vi "Stop Cooking.vi"(8 "error in (no error)":errorcluster, 11 "Cooker Actor in":refnum<class "Cooker Actor.lvclass">) -> (0 "error out":errorcluster, 3 "Cooker Actor out":refnum<class "Cooker Actor.lvclass">)   [LabVIEW 2021, in "Cooker Actor.lvlib" / "Cooker Actor.lvclass"]
uses:
  Cooker Actor.lvclass
  Oven Actor/Oven Actor Messages/Stop Heat Msg/Stop Heat Msg.lvclass
  <vilib>/ActorFramework/Actor/Actor.lvclass
  Cooker Actor Messages/Update Cooker Duration Msg/Update Cooker Duration Msg.lvclass
  Kitchen Actor Messages/Dye Whole Recipe Table Msg/Dye Whole Recipe Table Msg.lvclass
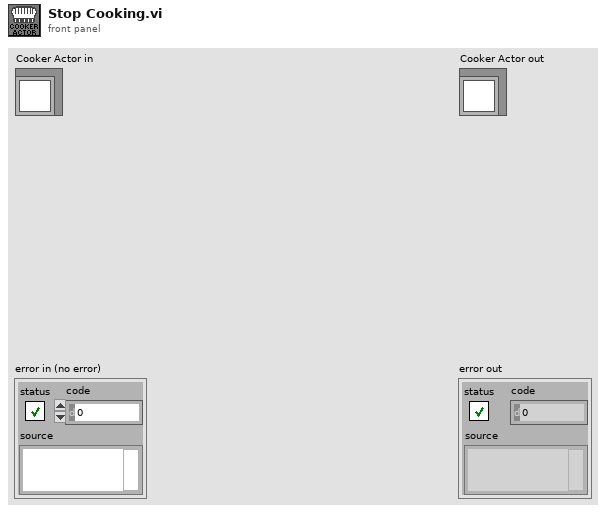
[diagram p1: front panel]
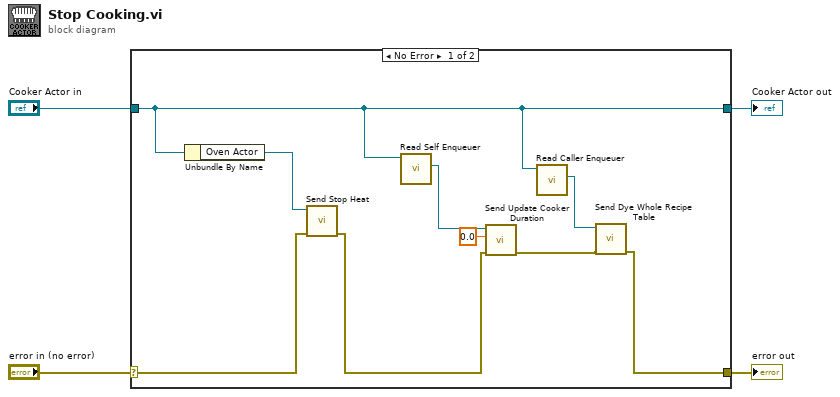
[diagram p0: block diagram]
diagram:
  n1 = case shown="No Error" "error in (no error)" {
    selector: "error in (no error)" -> [w12 w15]
    tunnel: [w5 w15] -> w3
    tunnel: [w8 w14] -> w1
    tunnel: "Cooker Actor in" -> [w8 w14]
    frame No Error {
      n2 = Unbundle By Name(w8) -> ("Oven Actor"=w13:refnum<class "Message Enqueuer.lvclass">)
      n3 = call "Send Stop Heat.vi"("error in (no error)"=w12, "Message Enqueuer"=w13) -> ("error out"=w9:errorcluster)  [unwired: 8 in, 1 out]
      n4 = call <vilib>:"Read Self Enqueuer.vi"("Actor"=w8) -> ("Self Enqueuer"=w11:refnum<class "Message Enqueuer.lvclass">)  [unwired: 10 in]
      n5 = call "Send Update Cooker Duration.vi"("error in (no error)"=w9, "Duration (s)"=0.0, "Message Enqueuer"=w11) -> ("error out"=w6:errorcluster)  [unwired: 7 in, 1 out]
      n6 = call <vilib>:"Read Caller Enqueuer.vi"("Actor"=w8) -> ("Caller Enqueuer"=w7:refnum<class "Message Enqueuer.lvclass">)  [unwired: 10 in]
      n7 = call "Send Dye Whole Recipe Table.vi"("error in (no error)"=w6, "Message Enqueuer"=w7) -> ("error out"=w5:errorcluster)  [unwired: 8 in, 1 out]
    }
    frame Error {
    }
  }
  "error out" <- w3
  "Cooker Actor out" <- w1
